vi "XLP80_Action_CANWriteA.vi"(7 "Function":string, 8 "err in":errorcluster) -> (0 "err out":errorcluster, 4 "WriteA Info":T1 {"WriteA Min" format="%.2f"; "WriteA Max" format="%.2f"})   [LabVIEW 2021]
uses:
  XLP80_Globals/XLP80_Globals_Referenzen.vi
  XLP80_Globals/Globals_Settings_XLP80.vi
  XLP80_Globals/XLP80_CAN_Globals.vi
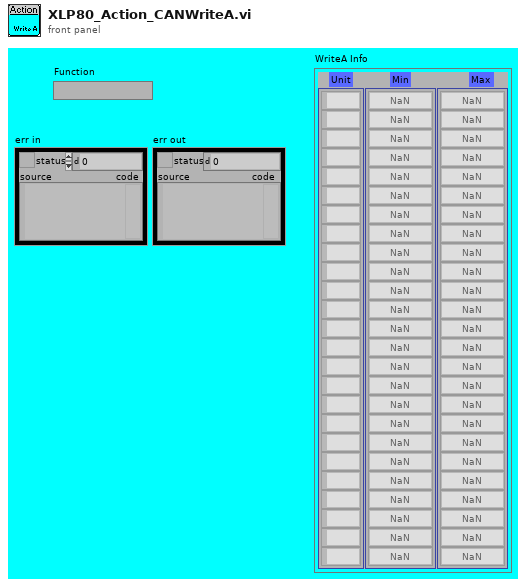
[diagram p1: front panel]
types:
  T1 = cluster{"WriteA Max":dbl[], "WriteA Min":dbl[], "WriteA Unit":string[]}
  T2 = cluster{"Signal Name":string[], "Description":string[], "Unit":string[], "Default":dbl[], "Min":dbl[], "Max":dbl[], "TestmodeA":bool[], "LogEnable":bool[]}
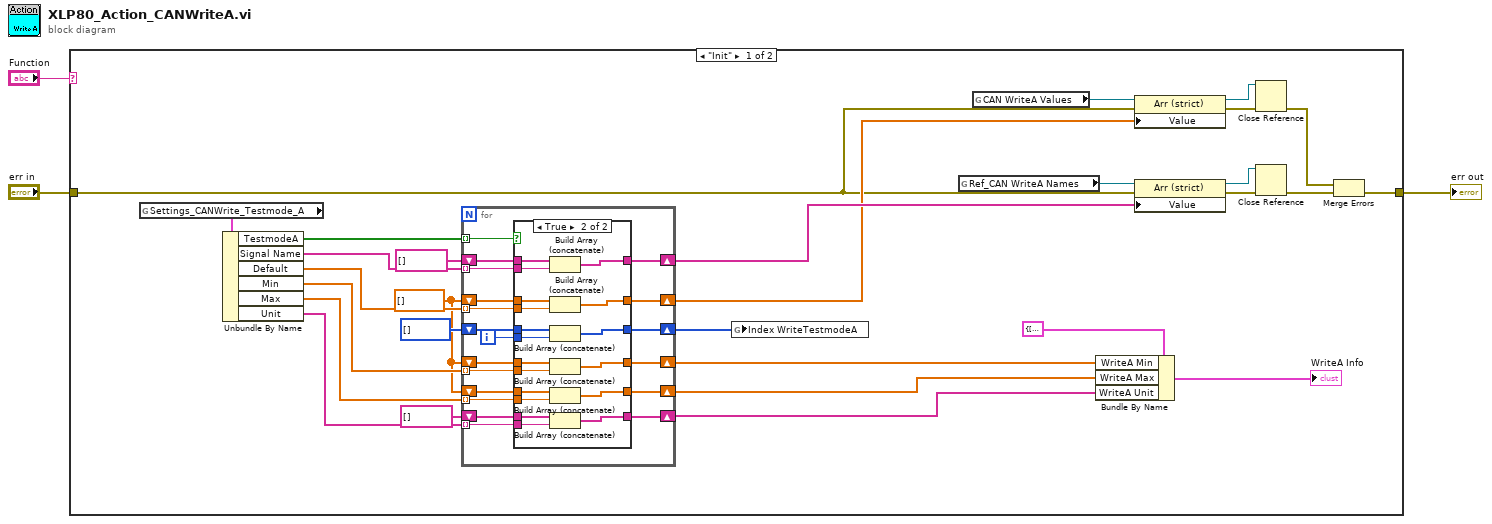
[diagram p0: block diagram]
diagram:
  n1 = case shown="\"Init\"" "Function" {
    tunnel: "err in" -> [w15 w76]
    tunnel: [w19 w76] -> w2
    frame "Init" {
      w5 = dbl[] [] ("Default")
      n2 = global read "Globals_Settings_XLP80.vi" "Settings_CANWrite_Testmode_A"() -> (w14:T2)
      n3 = Unbundle By Name(w14) -> ("TestmodeA"=w24:bool[], "Signal Name"=w27:string[], "Default"=w17:dbl[], "Min"=w13:dbl[], "Max"=w12:dbl[], "Unit"=w11:string[])
      n4 = for {
        tunnel: w24 -> [w51] mode=indexing
        shift-right: [w48] -> w23
        shift-left: string[] [] ("Signal Name") -> [w50]
        shift-right: [w45] -> w25
        shift-left: i32[] [] -> [w47]
        tunnel: w27 -> [w49] mode=indexing
        shift-right: [w42] -> w16
        shift-left: w5 -> [w44]
        tunnel: w17 -> [w43] mode=indexing
        tunnel: w13 -> [w41] mode=indexing
        tunnel: w12 -> [w40] mode=indexing
        tunnel: w11 -> [w39] mode=indexing
        shift-right: [w38] -> w7
        shift-left: string[] [] -> [w33]
        shift-right: [w37] -> w8
        shift-left: w5 -> [w34]
        shift-right: [w36] -> w9
        shift-left: w5 -> [w35]
        i -> [w46]
        n5 = case shown="True" w51 {
          tunnel: w50 -> [w57 w75]
          tunnel: w49 -> [_ w74]
          tunnel: [w57 w73] -> w48
          tunnel: w47 -> [w56 w72]
          tunnel: w46 -> [_ w71]
          tunnel: [w56 w70] -> w45
          tunnel: w44 -> [w55 w69]
          tunnel: w43 -> [_ w68]
          tunnel: [w55 w67] -> w42
          tunnel: w41 -> [_ w66]
          tunnel: w40 -> [_ w65]
          tunnel: w39 -> [_ w64]
          tunnel: [w52 w63] -> w38
          tunnel: [w53 w62] -> w37
          tunnel: [w54 w61] -> w36
          tunnel: w35 -> [w54 w60]
          tunnel: w34 -> [w53 w58]
          tunnel: w33 -> [w52 w59]
          frame False {
          }
          frame True {
            n6 = Build Array (concatenate)(w75, w74) -> (w73:string[])
            n7 = Build Array (concatenate)(w69, w68) -> (w67:dbl[])
            n8 = Build Array (concatenate)(w72, w71) -> (w70:i32[])
            n9 = Build Array (concatenate)(w60, w66) -> (w61:dbl[])
            n10 = Build Array (concatenate)(w58, w65) -> (w62:dbl[])
            n11 = Build Array (concatenate)(w59, w64) -> (w63:string[])
          }
        }
      }
      n12 = global write "XLP80_CAN_Globals.vi" "Index WriteTestmodeA"(w25) -> ()
      n13 = global read "XLP80_Globals_Referenzen.vi" "Ref_CAN WriteA Names"() -> (w30:refnum<vi>)
      n14 = global read "XLP80_Globals_Referenzen.vi" "CAN WriteA Values"() -> (w20:refnum<vi>)
      n15 = Bundle By Name(cluster=T1 {"WriteA Max"=[0.0, 0.0, 0.0, 0.0, 0.0, 0.0, 0.0, 0.0, 0.0, 0.0, 0.0, 0.0, 0.0, 0.0, 0.0, 0.0, 0.0, 0.0, 0.0, 0.0, 0.0, 0.0, 0.0, 0.0, 0.0, 0.0, 0.0, 1.0, 0.0, 0.0, 1.0], "WriteA Min"=[0.0, 0.0, 0.0, 0.0, 0.0, 0.0, 0.0, 0.0, 0.0, 0.0, 0.0, 0.0, 0.0, 0.0, 0.0, 0.0, 0.0, 0.0, 0.0, 0.0, 0.0, 0.0, 0.0, 0.0, 0.0, 0.0, 0.0, 1.0, 0.0, 0.0, 1.0], "WriteA Unit"=["", "", "", "", "", "", "", "", "", "", "", "", "", "", "", "", "", "", "", "", "", "", "", "", "", "", "", "", "", "", ""]} ("WriteA Info"), "WriteA Min"=w9, "WriteA Max"=w8, "WriteA Unit"=w7) -> (→"WriteA Info":T1)
      n16 = property class="Arr (strict)"(reference=w20, error in=w15, "Value"=w16) -> (reference out=w22:refnum<vi>, error out=w21:errorcluster)
      n17 = property class="Arr (strict)"(reference=w30, error in=w15, "Value"=w23) -> (reference out=w31:refnum<vi>, error out=w32:errorcluster)
      n18 = Close Reference(reference=w22, error in (no error)=w21) -> (error out=w18:errorcluster)
      n19 = Close Reference(reference=w31, error in (no error)=w32) -> (error out=w29:errorcluster)
      n20 = Merge Errors(w18, w29) -> (w19:errorcluster)
    }
    frame Default {
    }
  }
  "err out" <- w2
